vi "E08_FórmulaHerón.vi"() -> ()   [LabVIEW 2026]
panel:
  out "output variable":dbl
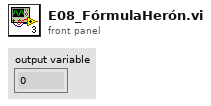
[diagram p1: front panel]
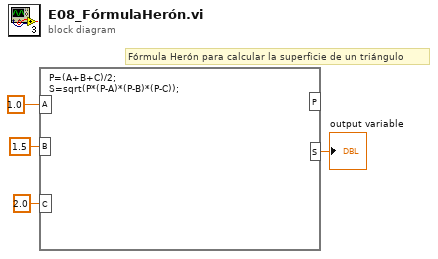
[diagram p0: block diagram]
diagram:
  # "Fórmula Herón para calcular la superficie de un triángulo"
  n1 = formula code="P=(A+B+C)/2;\nS=sqrt(P*(P-A)*(P-B)*(P-C));"("A"=1.0 ("input variable"), "B"=1.5 ("input variable"), "C"=2.0 ("input variable")) -> ("S"=→"output variable":dbl)  [unwired: 1 out]
